vi "changeSwitch.vi"(2 "数值":dbl=1.0 min=1.0 max=31.0 step=1.0, 3 "单片机串口":refnum<visa-resource-name>) -> (0 "返回值":string, 1 "单片机串口 2":refnum<visa-resource-name>)   [LabVIEW 2018]
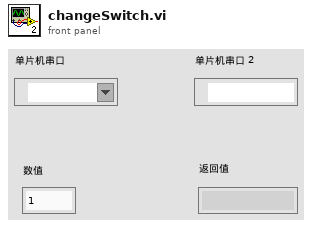
[diagram p1: front panel]
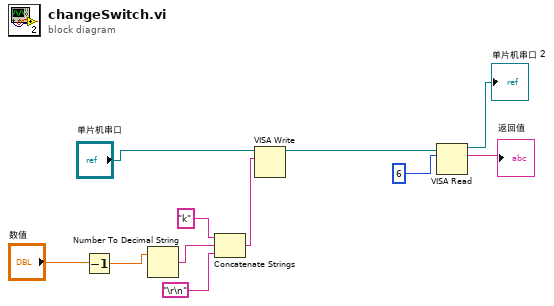
[diagram p0: block diagram]
diagram:
  n1 = Decrement(x="数值") -> (x-1=w5:dbl)
  n2 = Number To Decimal String(number=w5) -> (decimal integer string=w4:string)  [unwired: 1 in]
  n3 = Concatenate Strings("k", w4, "\r\n") -> (w8:string)
  n4 = VISA Write(VISA resource name="单片机串口", write buffer=w8) -> (VISA resource name out=w3:refnum<visa-resource-name>)  [unwired: 1 in, 2 out]
  n5 = VISA Read(VISA resource name=w3, byte count=6) -> (VISA resource name out=→"单片机串口 2":refnum<visa-resource-name>, read buffer=→"返回值":string)  [unwired: 1 in, 2 out]
